vi "PH_Tektronix_7000.set Trigger GUI Element.vi"(2 "Ref Trigger Config":refnum<vi>, 3 "Trigger Config":T1 {"Trigger Mode" items=["Normal", "Auto"]; "Coupling" items=["DC", "AC", "Hf Reject", "Lf Reject", "Noise Rej", "Atrigger"]; "Slope" items=["Rise", "Fall", "Either"]; "Source" items=["Channel1"=0, "Channel2"=1, "Channel3"=2, "Channel4"=3, "Aux"=12, "Line"=13]}, 4 "Enabled?":bool, 5 "error in":errorcluster) -> (19 "error out":errorcluster)   [LabVIEW 2014, in "PH_Tektronix_7000.lvlib"]
doc: "If the reference is valid, the incoming data are set to the GUI."
uses:
  PH_Tektronix_7000.lvlib
  PH_Tektronix_7000.Trigger Config.ctl
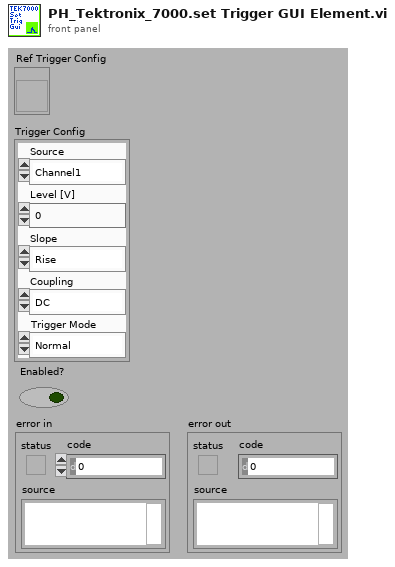
[diagram p1: front panel]
types:
  T1 = typedef "PH_Tektronix_7000.lvlib/PH_Tektronix_7000.Trigger Config.ctl" = cluster{"Source":u16, "Level [V]":dbl, "Slope":u16, "Coupling":u16, "Trigger Mode":u16}
  T2 = enum8{"Enabled", "Disabled", "Disabled and Grayed Out"}
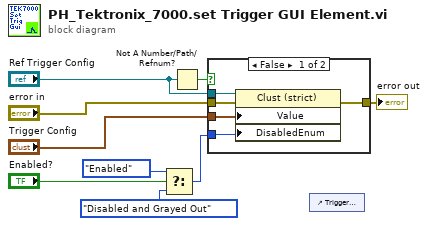
[diagram p0: block diagram]
diagram:
  n1 = Select(t=T2."Enabled" ("Disabled"), s="Enabled?", f=T2."Disabled and Grayed Out") -> (s? t:f=w4:T2)
  n2 = Not A Number/Path/Refnum?(number/path/refnum="Ref Trigger Config") -> (NaN/Path/Refnum?=w9:bool)
  n3 = case shown="False" w9 {
    tunnel: "error in" -> [w14 w15]
    tunnel: [w13 w15] -> w7
    tunnel: "Ref Trigger Config" -> [w12 _]
    tunnel: "Trigger Config" -> [w11 _]
    tunnel: w4 -> [w10 _]
    frame False {
      n4 = property class="Clust (strict)"(reference=w12, error in=w14, "Value"=w11, "DisabledEnum"=w10) -> (error out=w13:errorcluster)  [unwired: 1 out]
    }
    frame True {
    }
  }
  "error out" <- w7
  n5 = control-ref of="Trigger Config"() -> ()  [unwired: 1 out]
